vi "Configure Color Grade.vi"(0 "VISA resource name":refnum<visa-resource-name>, 1 "Duty Cycle Distortion Format (0: Time)":i32(ring) items=["Time", "Percent"], 5 "Measurement Type (0: Crossing Level Percent)":i32(ring) items=["Crossing Level Percent", "Duty Cycle Distortion", "Eye Height", "Eye Width", "Jitter", "Q Factor"], 7 "Measurement Source (0: Channel 1)":i32(ring) items=["Channel 1", "Channel 2", "Channel 3", "Channel 4", "Common 1", "Common 2", "Differential 1", "Differential 2", "Memory 1", "Memory 2", "Memory 3", "Memory 4", "Function 1", "Function 2", "Function 3", "Function 4", "Function 5", "Function 6", "Function 7", "Function 8", "Function 9", "Function 10", "Function 11", "Function 12", "Function 13", "Function 14", "Function 15", "Function 16", "Clock", "Equalized", "MTRend", "MSPectrum"], 9 "Algorithm (1: Extrapolated)":i32(ring)=1 items=["Measured", "Extrapolated"], 11 "error in (no error)":errorcluster, 12 "Jitter Format (0: PP)":i32(ring) items=["PP", "RMS"]) -> (4 "VISA resource name out":refnum<visa-resource-name>, 15 "error out":errorcluster)   [LabVIEW 2020, in "Agilent 90000 Series.lvlib"]
doc: "Configures the color grade's parameters.\n\n<b>Notes:</b> \n1. This VI is new in firmware version 5.00\n2. Before using this command or query, you must use the :DISPlay:CGRade command to enable the color grade persistence feature."
uses:
  Agilent 90000 Series.lvlib
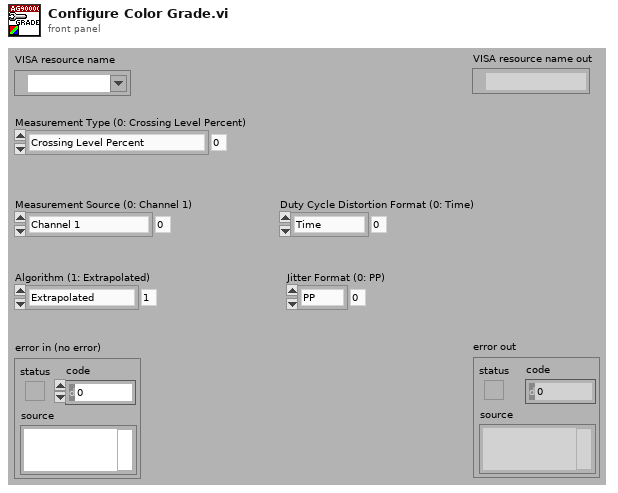
[diagram p1: front panel]
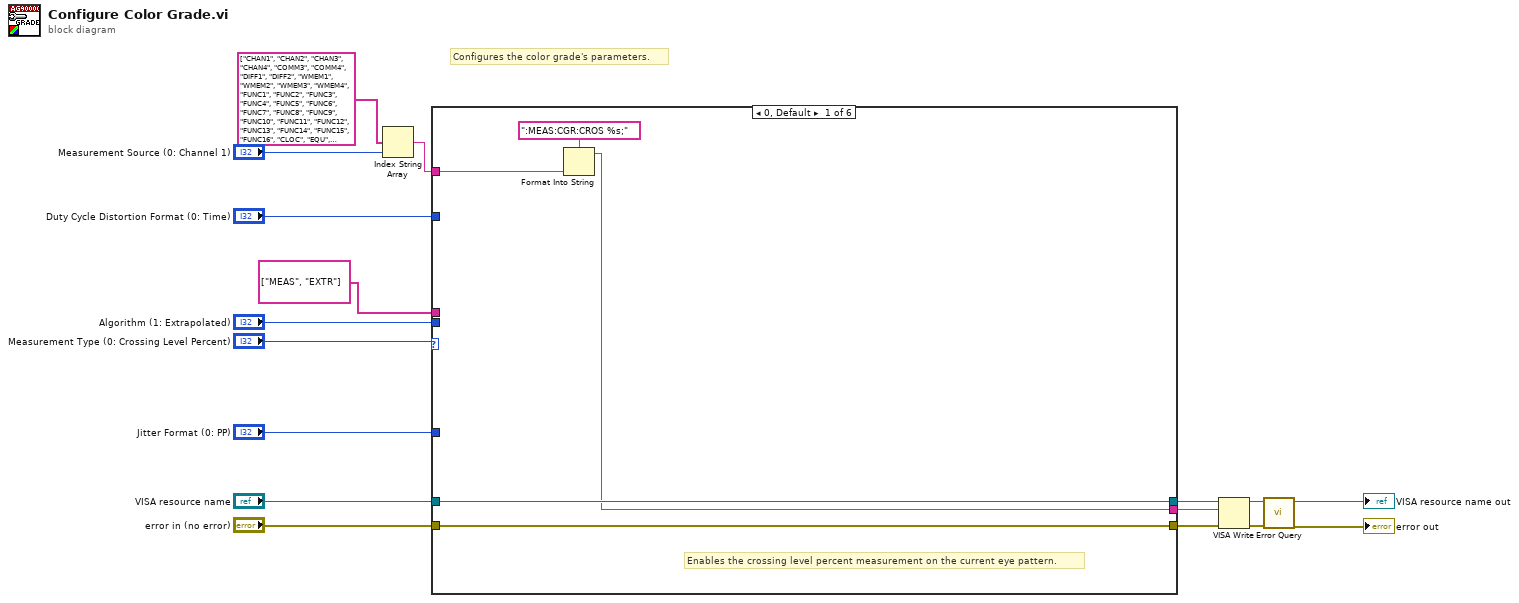
[diagram p0: block diagram]
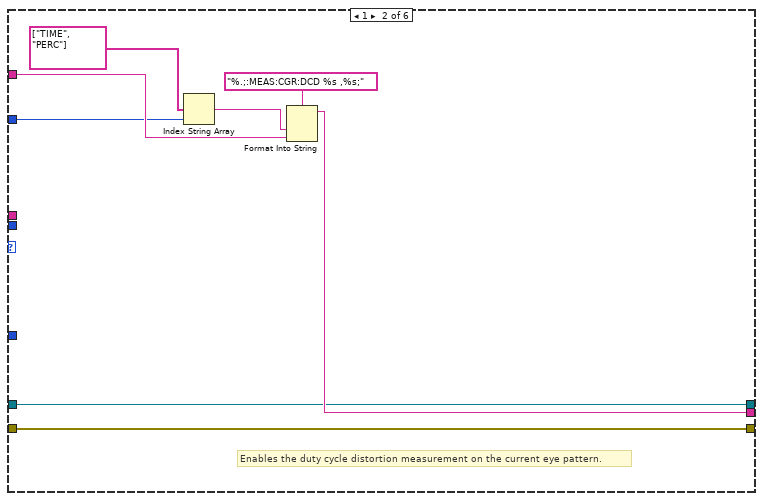
[diagram p2: hidden frame]
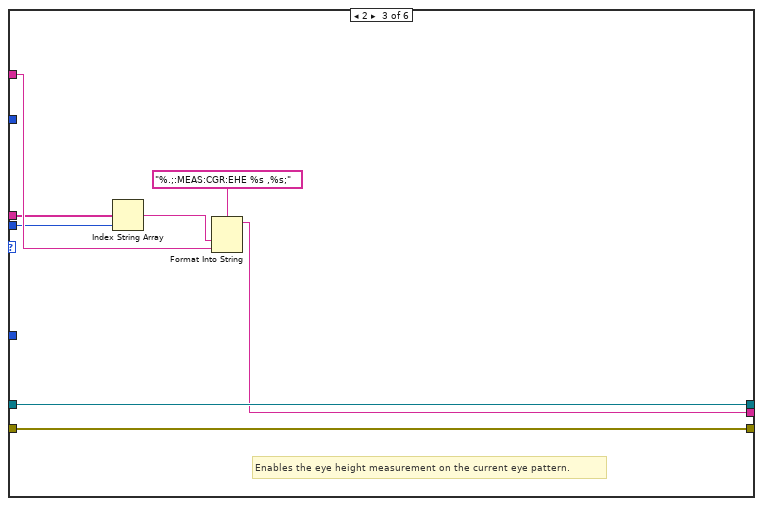
[diagram p3: hidden frame]
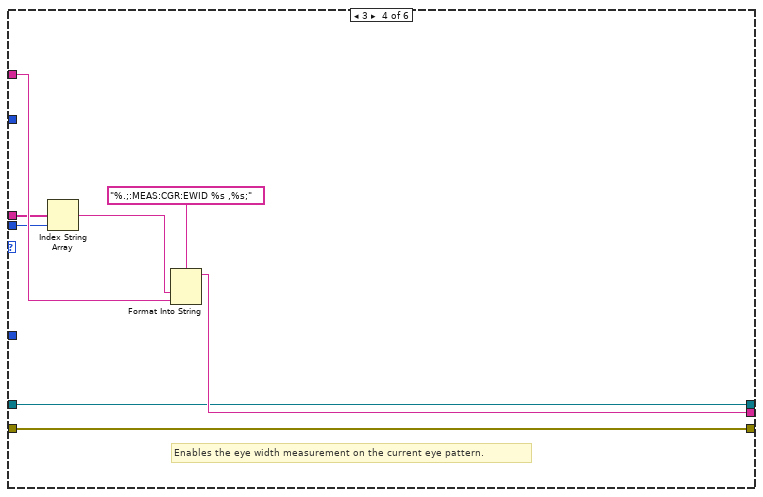
[diagram p4: hidden frame]
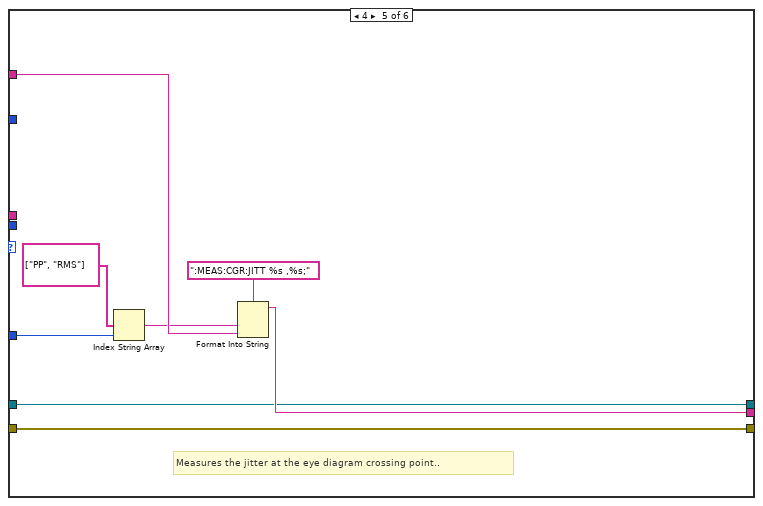
[diagram p5: hidden frame]
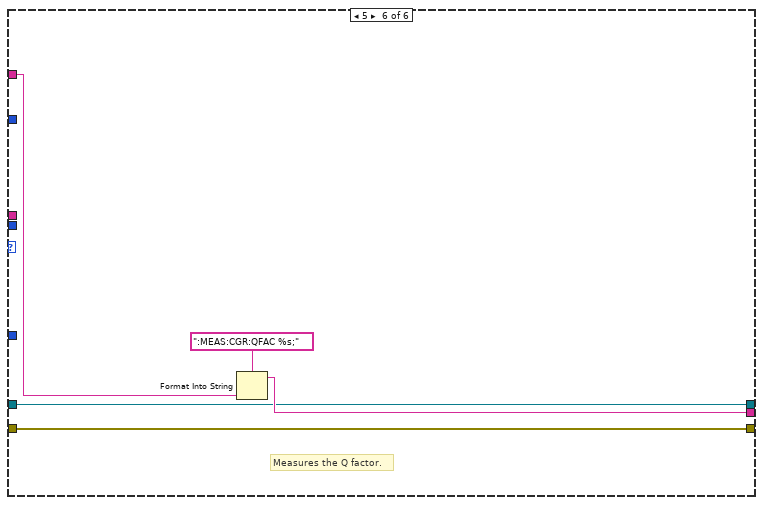
[diagram p6: hidden frame]
diagram:
  # "Configures the color grade's parameters."
  n1 = Index String Array(1:"Measurement Source (0: Channel 1)", 2:string[] ["CHAN1", "CHAN2", "CHAN3", "CHAN4", "COMM3", "COMM4", "DIFF1", "DIFF2", "WMEM1", "WMEM2", "WMEM3", "WMEM4", "FUNC1", "FUNC2", "FUNC3", "FUNC4", "FUNC5", "FUNC6", "FUNC7", "FUNC8", "FUNC9", "FUNC10", "FUNC11", "FUNC12", "FUNC13", "FUNC14", "FUNC15", "FUNC16", "CLOC", "EQU", "MTR", "MSP"] ("subarray 2")) -> (0:w16:string)  [unwired: 1 in]
  n2 = case shown="0, Default" "Measurement Type (0: Crossing Level Percent)" {
    tunnel: w16 -> [w21 w29 w37 w45 w53 w58]
    tunnel: "VISA resource name" -> [w20 w27 w36 w43 w51 w56]
    tunnel: [w20 w27 w36 w43 w51 w56] -> w10
    tunnel: "error in (no error)" -> [w19 w26 w35 w42 w50 w55]
    tunnel: [w19 w26 w35 w42 w50 w55] -> w8
    tunnel: [w18 w28 w34 w44 w52 w57] -> w7
    tunnel: string[] ["MEAS", "EXTR"] ("string array") -> [_ _ w33 w41 _ _]
    tunnel: "Duty Cycle Distortion Format (0: Time)" -> [_ w25 _ _ _ _]
    tunnel: "Algorithm (1: Extrapolated)" -> [_ _ w32 w40 _ _]
    tunnel: "Jitter Format (0: PP)" -> [_ _ _ _ w48 _]
    frame 0, Default {
      # "Enables the crossing level percent measurement on the current eye pattern."
      n3 = Format Into String(format string=":MEAS:CGR:CROS %s;", w21) -> (resulting string=w18:string)  [unwired: 2 in, 1 out]
    }
    frame 1 {
      # "Enables the duty cycle distortion measurement on the current eye pattern."
      n4 = Index String Array(1:w25, 2:string[] ["TIME", "PERC"] ("string array")) -> (0:w24:string)  [unwired: 1 in]
      n5 = Format Into String(format string="%.;:MEAS:CGR:DCD %s ,%s;", w24, w29) -> (resulting string=w28:string)  [unwired: 2 in, 1 out]
    }
    frame 2 {
      # "Enables the eye height measurement on the current eye pattern."
      n6 = Index String Array(1:w32, 2:w33) -> (0:w31:string)  [unwired: 1 in]
      n7 = Format Into String(format string="%.;:MEAS:CGR:EHE %s ,%s;", w31, w37) -> (resulting string=w34:string)  [unwired: 2 in, 1 out]
    }
    frame 3 {
      # "Enables the eye width measurement on the current eye pattern."
      n8 = Index String Array(1:w40, 2:w41) -> (0:w39:string)  [unwired: 1 in]
      n9 = Format Into String(format string="%.;:MEAS:CGR:EWID %s ,%s;", w39, w45) -> (resulting string=w44:string)  [unwired: 2 in, 1 out]
    }
    frame 4 {
      # "Measures the jitter at the eye diagram crossing point.."
      n10 = Index String Array(1:w48, 2:string[] ["PP", "RMS"] ("string array")) -> (0:w47:string)  [unwired: 1 in]
      n11 = Format Into String(format string=":MEAS:CGR:JITT %s ,%s;", w47, w53) -> (resulting string=w52:string)  [unwired: 2 in, 1 out]
    }
    frame 5 {
      # "Measures the Q factor."
      n12 = Format Into String(format string=":MEAS:CGR:QFAC %s;", w58) -> (resulting string=w57:string)  [unwired: 2 in, 1 out]
    }
  }
  n13 = VISA Write(VISA resource name=w10, write buffer=w7, error in (no error)=w8) -> (VISA resource name out=w15:refnum<visa-resource-name>, error out=w14:errorcluster)  [unwired: 1 out]
  n14 = call "Error Query.vi"("error in (no error)"=w14, "VISA resource name"=w15) -> ("error out"=→"error out":errorcluster, "VISA resource name out"=→"VISA resource name out":refnum<visa-resource-name>)  [unwired: 6 in, 2 out]
